vi "TypeDef Demo.vi"() -> ()   [LabVIEW 2014]
uses:
  Controls/Strict TypeDef.ctl
  Controls/TypeDef.ctl
panel:
  in  "TypeDef":T1
  in  "Strict TypeDef":T2
  in  "Custom Control":cluster{"Numeric Control":dbl, "String":string}
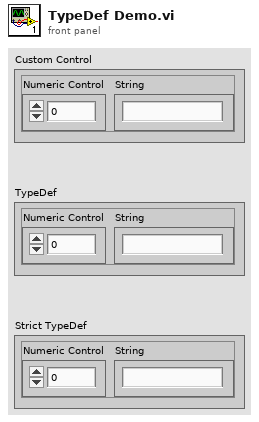
[diagram p1: front panel]
types:
  T1 = typedef "TypeDef.ctl" = cluster{"Numeric Control":dbl, "String":string}
  T2 = typedef "Strict TypeDef.ctl" = cluster{"Numeric Control":dbl, "String":string}
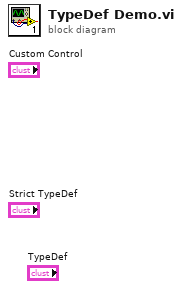
[diagram p0: block diagram]
diagram:
